vi "Longitudinal-Radial Distance_2011.vi"(3 "Image (Counts)":dbl[][](array[numeric]), 4 "ROI infos":T3={"npix-X"=512, "npix-Y"=384, "Left [pix]"=0.0, "Top [pix]"=0.0}, 5 "Screen&Camera":T1={"Screen Orientation"="Regular", "Screen angle"="Flat", "Lens"=enum."FL1-f8x08", "Calibration (mm/pix)"=1.0}) -> (0 "Z map":dbl[][](array[numeric]), 2 "R^2 map":dbl[][](array[numeric]))   [LabVIEW 2013]
uses:
  SubVis/ScreenCam2_TypDEf.ctl
  SubVis/CamAndObj_TypDEf.ctl
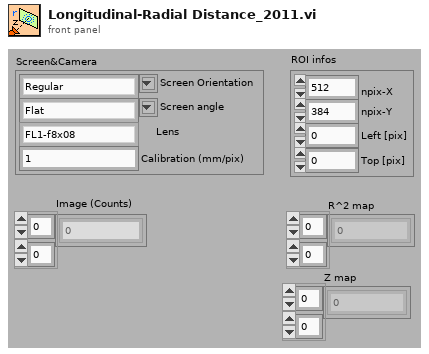
[diagram p1: front panel]
types:
  T1 = typedef "ScreenCam2_TypDEf.ctl" = cluster{"Screen Orientation":string, "Screen angle":string, "Lens":T2, "Calibration (mm/pix)":dbl}
  T2 = typedef "CamAndObj_TypDEf.ctl" = enum16{"FL1-f8x08", "FL1-f8x06", "FL1-f8", "ch300-f50", "FL2G-f8", "FL3M14-f8", "FL3M14-f8x08", "FL3M14-f8x08(2x2)"}
  T3 = cluster{"npix-X":i32, "npix-Y":i32, "Left [pix]":dbl, "Top [pix]":dbl}
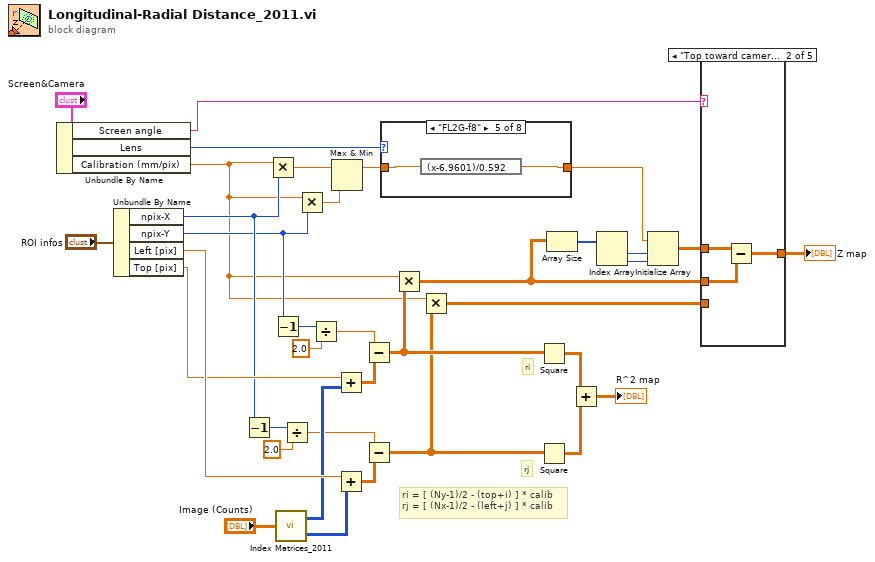
[diagram p0: block diagram]
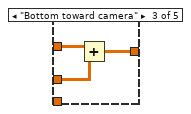
[diagram p3: hidden frame]
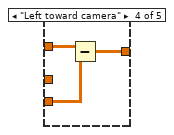
[diagram p4: hidden frame]
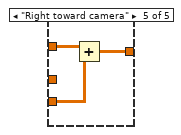
[diagram p5: hidden frame]
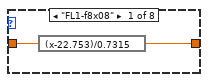
[diagram p6: hidden frame]
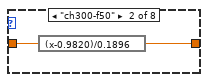
[diagram p7: hidden frame]
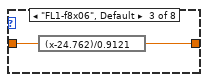
[diagram p8: hidden frame]
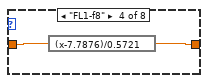
[diagram p9: hidden frame]
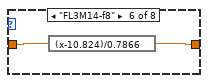
[diagram p10: hidden frame]
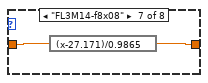
[diagram p11: hidden frame]
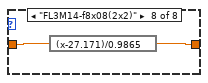
[diagram p12: hidden frame]
diagram:
  # "ri = [ (Ny-1)/2 - (top+i) ] * calib\nrj = [ (Nx-1)/2 - (left+j) ] * calib"
  # "ri"
  # "rj"
  n1 = Unbundle By Name("Screen&Camera") -> ("Screen angle"=w33:string, "Lens"=w36:T2, "Calibration (mm/pix)"=w3:dbl)
  n2 = Unbundle By Name("ROI infos") -> ("npix-X"=w20:i32, "npix-Y"=w19:i32, "Left [pix]"=w25:dbl, "Top [pix]"=w21:dbl)
  n3 = Decrement(x=w20) -> (x-1=w32:i32)
  n4 = Multiply(x=w3, y=w20) -> (x*y=w16:dbl)
  n5 = Decrement(x=w19) -> (x-1=w31:i32)
  n6 = call "Index Matrices_2011.vi"("Image In"="Image (Counts)") -> ("M(j)"=w24:i32[][], "M(i)"=w17:i32[][])  [unwired: 2 out]
  n7 = Divide(x=w32, y=2.0) -> (x/y=w12:dbl)
  n8 = Multiply(x=w3, y=w19) -> (x*y=w15:dbl)
  n9 = Divide(x=w31, y=2.0) -> (x/y=w13:dbl)
  n10 = Max & Min(x=w16, y=w15) -> (max(x,y)=w14:dbl)  [unwired: 1 out]
  n11 = Add(x=w21, y=w17) -> (x+y=w22:dbl[][])
  n12 = Add(x=w25, y=w24) -> (x+y=w23:dbl[][])
  n13 = Subtract(x=w13, y=w22) -> (x-y=w5:dbl[][])
  n14 = Subtract(x=w12, y=w23) -> (x-y=w4:dbl[][])
  n15 = case shown="\"FL2G-f8\"" w36 {
    tunnel: w14 -> [w38 w40 w42 w44 w46 w48 w50 w52]
    tunnel: [w37 w39 w41 w43 w45 w47 w49 w51] -> w8
    frame "FL1-f8x08" {
      n16 = expression code="(x-22.753)/0.7315"(w38) -> (w37:dbl)
    }
    frame "ch300-f50" {
      n17 = expression code="(x-0.9820)/0.1896"(w40) -> (w39:dbl)
    }
    frame "FL1-f8x06", Default {
      n18 = expression code="(x-24.762)/0.9121"(w42) -> (w41:dbl)
    }
    frame "FL1-f8" {
      n19 = expression code="(x-7.7876)/0.5721"(w44) -> (w43:dbl)
    }
    frame "FL2G-f8" {
      n20 = expression code="(x-6.9601)/0.592"(w46) -> (w45:dbl)
    }
    frame "FL3M14-f8" {
      n21 = expression code="(x-10.824)/0.7866"(w48) -> (w47:dbl)
    }
    frame "FL3M14-f8x08" {
      n22 = expression code="(x-27.171)/0.9865"(w50) -> (w49:dbl)
    }
    frame "FL3M14-f8x08(2x2)" {
      n23 = expression code="(x-27.171)/0.9865"(w52) -> (w51:dbl)
    }
  }
  n24 = Multiply(x=w3, y=w5) -> (x*y=w2:dbl[][])
  n25 = Multiply(x=w3, y=w4) -> (x*y=w1:dbl[][])
  n26 = Square(x=w5) -> (x^2=w27:dbl[][])
  n27 = Square(x=w4) -> (x^2=w28:dbl[][])
  n28 = Array Size(array=w2) -> (size(s)=w9:i32[])
  n29 = Add(x=w27, y=w28) -> (x+y=→"R^2 map":dbl[][])
  n30 = Index Array(array=w9) -> (element #1=w10:i32, element #2=w11:i32)  [unwired: 2 in]
  n31 = Initialize Array(w8, w10, w11) -> (w7:dbl[][])
  n32 = case shown="\"Top toward camera\"" w33 {
    tunnel: w7 -> [w53 w56 w59 w62 w65]
    tunnel: w2 -> [_ w55 w58 _ _]
    tunnel: w1 -> [_ _ _ w61 w64]
    tunnel: [w53 w54 w57 w60 w63] -> w6
    frame "Flat", Default {
    }
    frame "Top toward camera" {
      n33 = Subtract(x=w56, y=w55) -> (x-y=w54:dbl[][])
    }
    frame "Bottom toward camera" {
      n34 = Add(x=w59, y=w58) -> (x+y=w57:dbl[][])
    }
    frame "Left toward camera" {
      n35 = Subtract(x=w62, y=w61) -> (x-y=w60:dbl[][])
    }
    frame "Right toward camera" {
      n36 = Add(x=w65, y=w64) -> (x+y=w63:dbl[][])
    }
  }
  "Z map" <- w6
